vi "CN0u.vi"(1 "Uplink free space path loss (dB)":dbl, 2 "G/Tsat (dBK-1)":dbl, 3 "EIRP ground (dBW)":dbl) -> (0 "C/N0 uplink (dBHz)":dbl)   [LabVIEW 2015]
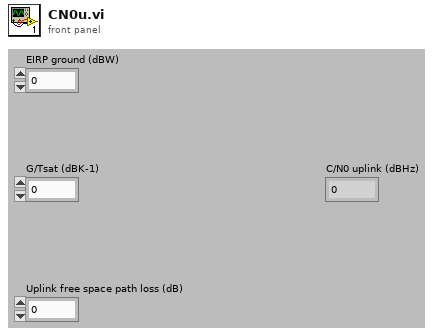
[diagram p1: front panel]
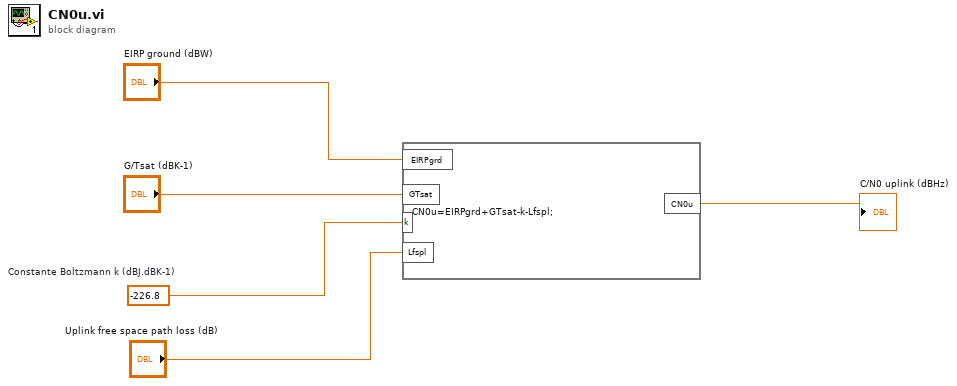
[diagram p0: block diagram]
diagram:
  w3 = -226.8  # Constante Boltzmann k (dBJ.dBK-1)
  n1 = formula code="CN0u=EIRPgrd+GTsat-k-Lfspl;"("EIRPgrd"="EIRP ground (dBW)", "GTsat"="G/Tsat (dBK-1)", "k"=w3, "Lfspl"="Uplink free space path loss (dB)") -> ("CN0u"=→"C/N0 uplink (dBHz)":dbl)
